vi "Test B.vi"(7 "Socket":i32, 8 "error in (no error)":errorcluster, 9 "b":dbl[](array[numeric])=[100.0, 100.0, 100.0], 10 "a":dbl[](array[numeric])=[0.0, 0.0, 0.0], 11 "x":dbl[](array[numeric])=[50.0, 51.0, 52.0]) -> (0 "error out":errorcluster)   [LabVIEW 2019, in "Multisocket Example(Station1).lvlib"]
uses:
  Multisocket Example(Station1).lvlib
  400e6fd7-5c57-4563-98c8-4c487ac03ebd.vi
  d135eecd-02d8-4d26-94c7-1196041114e8.vi
  LVUT Global 1.vi
  <vilib>/Utility/Data Type/Get Type Information.vi
  <vilib>/Utility/error.llb/Trim Whitespace.vi
  Almost Equal.vi
  Unit Test Engine Tools.lvlib
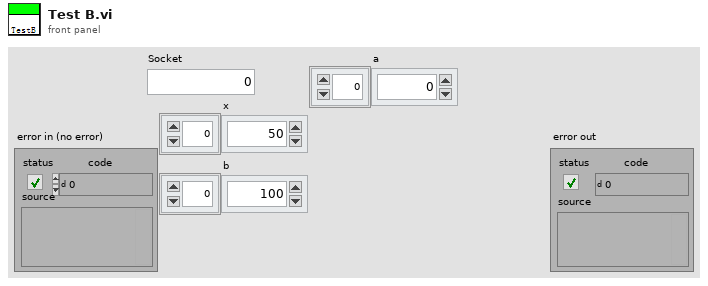
[diagram p1: front panel]
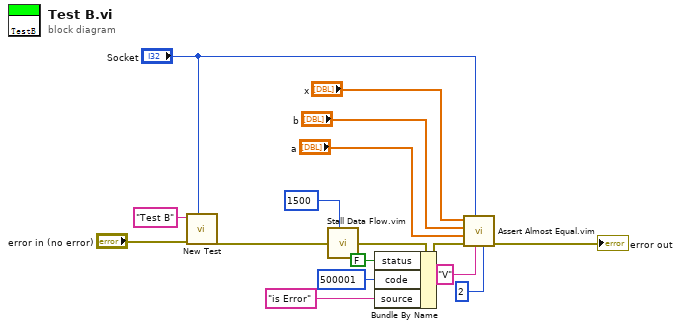
[diagram p0: block diagram]
diagram:
  n1 = call "New Test.vi"("Socket"="Socket", "error in (no error)"="error in (no error)", "Test"="Test B") -> ("error out"=w14:errorcluster)  [unwired: 8 in]
  n2 = call "Stall Data Flow.vim"("value in"=w14, "milliseconds to wait"=u32 1500) -> ("value out"=w11:errorcluster)  [unwired: 1 out]
  n3 = Bundle By Name(cluster=w11, "status"=FALSE, "code"=500001, "source"="is Error") -> (w6:errorcluster)
  n4 = call "Assert Almost Equal.vim"("precision (2)"=i16 2 ("precision (6)"), "Unit"="V", "Socket"="Socket", "error in (no error)"=w6, "a"="a", "b"="b", "x"="x") -> ("error out"=→"error out":errorcluster)  [unwired: 4 in]
